vi "RT Main v0.99.vi"() -> ()   [LabVIEW 2017]
doc: "Changelog:\n\nv0.9:\n- Autocycle"
uses:
  Controls/Auto Delays.ctl
  support/Controls/All Inputs.ctl
  support/Controls/Index Details.ctl
  support/Controls/Auto Stats.ctl
  Controls/Auto Times.ctl
  Global Variables/RT GV.vi
  support/Message Queue/Enqueue Message (Single).vi
  Global Variables/FPGA GV.vi
  <vilib>/Utility/error.llb/Error Cluster From Error Code.vi
  <vilib>/rvi/errors/niLvFpgaAdjustHostInterfaceError.vi
  Global Variables/Network Globals.vi
  <vilib>/FPGAPlugInAG/Dynamic/niLvFpga_Close_Dynamic.vi
  <vilib>/rvi/interface/nirviReadWriteControl/nirviReadWriteControl.xnode
  Controls/FPGA Ref.ctl
  <vilib>/rvi/interface/nirviCloseFPGA/nirviCloseFPGA.xnode
  support/Message Queue/Message Queue.lvlib
  NiFpgaLv.dll
  <vilib>/rvi/interface/Simulation/niFpgaSimulationCallBeginRW.vi
panel:
  in  "Auto Para":T1={"Agitator Delays"=[250, 350], "TF Delays"=[700, 800, 2], "Insertion Delays"=[100, 500], "Cutting Delays"=[300, 300, 100], "PF Delays"=[250, 30000], "Measur. Delays"=[500.0, 188.9, 1.0], "Reject Delays"=[500], "BF Delays"=[1000, 1000]}
  in  "Counts in":cluster{"OutputCount":u32, "RejectCount":u32}
  in  "Stop Button 4":bool
  out "error out":errorcluster
  out "Wrong Message":string
  in  "Stop Button":bool
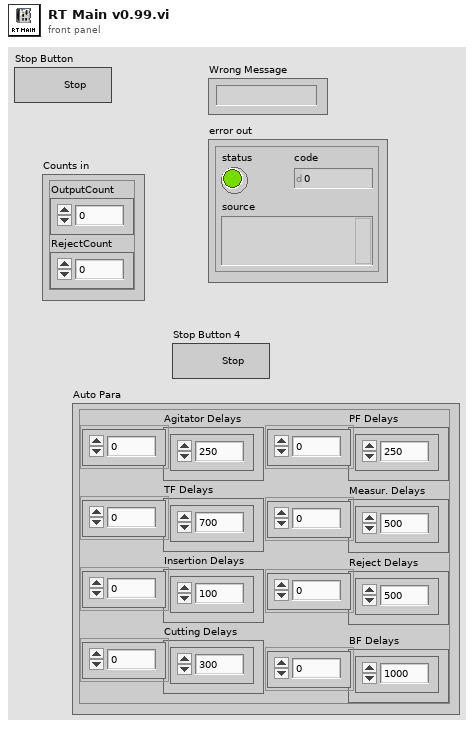
[diagram p1: front panel]
types:
  T1 = typedef "Auto Delays.ctl" = cluster{"Agitator Delays":u32[], "TF Delays":u32[], "Insertion Delays":u32[], "Cutting Delays":u32[], "PF Delays":u32[], "Measur. Delays":dbl[], "Reject Delays":u32[], "BF Delays":u32[]}
  T2 = typedef "FPGA Ref.ctl" = refnum<k20>
  T3 = cluster{"TL_Red":bool, "TL_Orange":bool, "TL_Green":bool, "TL_Buzzer":bool, "SOL_Index_Rotary_CW":bool, "SOL_Index_CNVR_Rotary_CCW":bool, "SOL_Index_CNVR_Stopper_Rear":bool, "SOL_Index_CNVR_Output _Separator _Rear":bool, "Bowl  Feeder_ ON":bool, "Pump_CNVR_Motor _ON":bool, "SOL_Gating_CYL_Rear":bool, "SOL_Tube_Feed_Agitatator":bool, "SOL_Tube_Feed_Gating_CYL":bool, "SOL_Insertion _CYL":bool, "SOL_Insertion_Clamp_CYL":bool, "SOL_Cutting_CYL":bool, "SOL_Cutting_Clamp_CYL":bool, "SOL_Insertion_Air_Nozzle":bool, "SOL_Measurement_CYL":bool, "SOL_Measure_Clamp_CYL":bool, "SOL_Rejection CYL_1":bool, "SOL_Rejection CYL_2":bool, "SOL_Rejection CYL_3":bool, "SOL_Rejection CYL_4":bool, "DO1.24":bool, "DO1.25":bool, "DO1.26":bool, "DO1.27":bool, "DO1.28":bool, "DO1.29":bool, "DO1.30":bool, "DO1.31":bool}
  T4 = typedef "All Inputs.ctl" = cluster{"DI 1":cluster{"Machine_ON":bool, "E_stop ":bool, "SW_Pressure":bool, "SW_Start ":bool, "SW_Reset":bool, "SW_Stop":bool, "SW_Door":bool, "RS_Index_Rotary_CW":bool, "RS_Index_Rotary_CCW":bool, "RS_Index_Stopper _Rear":bool, "RS_Index_Output_Separator_Rear":bool, "PES_Index_Pallet_Sensor":bool, "PES_Index_Output_Part Sensor":bool, "ICS_BF_Low_Level_1":bool, "ICS_BF_Low_Level_2":bool, "ICS_BF_Pump_CNVR_Full_1":bool, "ICS_BF_Pump_CNVR_Full_2":bool, "ICS_BF_Pump_CNVR_Full_3":bool, "ICS_BF_Pump_CNVR_Full_4":bool, "PES_PC_Pump Presence_1":bool, "PES_PC_Pump Presence_2":bool, "PES_PC_Pump Presence_3":bool, "PES_PC_Pump Presence_4":bool, "RS_PC_Gating_Front":bool, "PES_Pump_Interference":bool, "PES_TF_Low_Level":bool, "PES_Tube Presence_1":bool, "PES_Tube Presence_2":bool, "PES_Tube Presence_3":bool, "PES_Tube Presence_4":bool, "DI1.30":bool, "DI1.31":bool}, "DI 2":cluster{"RS_Agitatator_1_Rear ":bool, "RS_Agitatator_2_Rear ":bool, "RS_TF_Gating CYL_Rear":bool, "RS_Insertion_1_Rear":bool, "RS_Insertion_1_Front":bool, "RS_Insertion _2_Rear":bool, "RS_Insertion _2_Front":bool, "RS_Insertion _3_Rear":bool, "RS_Insertion _3_Front":bool, "RS_Insertion _4_Rear":bool, "RS_Insertion _4_Front":bool, "RS_Insertion_Clamp_Rear":bool, "RS_Cutting_Rear":bool, "RS_Cutting_Clamp _Rear":bool, "RS_Measurement_1_Rear":bool, "RS_Measurement_2_Rear":bool, "RS_Measurement_3_Rear":bool, "RS_Measurement_4_Rear":bool, "RS_Measure_Clamp_Rear":bool, "RS_Rejection_1_Rear":bool, "RS_Rejection_2_Rear":bool, "RS_Rejection_3_Rear":bool, "RS_Rejection_4_Rear":bool, "DI2.23":bool, "DI2.24":bool, "DI2.25":bool, "DI2.26":bool, "DI2.27":bool, "DI2.28":bool, "DI2.29":bool, "DI2.30":bool, "DI2.31":bool}, "IAS 1":dbl, "IAS 2":dbl, "IAS 3":dbl, "IAS 4":dbl, "DO 1":cluster{"TL_Red":bool, "TL_Orange":bool, "TL_Green":bool, "TL_Buzzer":bool, "SOL_Index_Rotary_CW":bool, "SOL_Index_CNVR_Rotary_CCW":bool, "SOL_Index_CNVR_Stopper_Rear":bool, "SOL_Index_CNVR_Output _Separator _Rear":bool, "Bowl  Feeder_ ON 1":bool, "Pump_CNVR_Motor _ON":bool, "SOL_PC_Gating_CYL_Rear":bool, "SOL_Tube_Feed_Agitatator":bool, "SOL_Tube_Feed_Gating_CYL":bool, "SOL_Insertion _CYL":bool, "SOL_Insertion_Clamp_CYL":bool, "SOL_Cutting_CYL":bool, "SOL_Cutting_Clamp_CYL":bool, "SOL_Insertion_Air_Nozzle":bool, "SOL_Measurement_CYL":bool, "DO1.19":bool, "SOL_Rejection CYL_1":bool, "SOL_Rejection CYL_2":bool, "SOL_Rejection CYL_3":bool, "SOL_Rejection CYL_4":bool, "Bowl  Feeder_ ON 2":bool, "SOL_BF_BlowerON":bool, "SOL_BF1_Track1":bool, "SOL_BF1_Track2":bool, "SOL_BF2_Track1":bool, "SOL_BF2_Track2":bool, "DO1.30":bool, "DO1.31":bool}}
  T5 = typedef "Index Details.ctl" = cluster{"Time (ms)":u32, "Waveform Graph":i16[]}
  T6 = cluster{T1, "Reject Pallets":cluster{"Reject 1":bool, "Reject 2":bool, "Reject 3":bool, "Reject 4":bool}}
  T7 = typedef "Auto Stats.ctl" = cluster{"Time":timestamp, "OEE":cluster{"AVL":dbl, "PRF":dbl, "QUA":dbl, "OEE":dbl}, "Auto Times":T8, "Counts out":cluster{"OutputCount":u32, "RejectCount":u32}, "Measurements":cluster{"1":dbl, "2":dbl, "3":dbl, "4":dbl}, "Outputs":cluster{"OutputCount":u32, "Numeric Control":u32}}
  T8 = typedef "Auto Times.ctl" = cluster{"Index Time":u32, "TF Time":u32, "Insertion Time":u32, "Cutting Time":u32, "PF Time":u32, "Meas. Time":u32, "Reject Time":u32}
  T9 = cluster{string, dbl, "Counts in":cluster{"OutputCount":u32, "RejectCount":u32}, "Auto Para":T1}
  T10 = cluster{"TL_Red":bool, "TL_Orange":bool, "TL_Green":bool, "TL_Buzzer":bool, "SOL_Index_Rotary_CW":bool, "SOL_Index_CNVR_Rotary_CCW":bool, "SOL_Index_CNVR_Stopper_Rear":bool, "SOL_Index_CNVR_Output _Separator _Rear":bool, "Bowl Feeder_ ON1":bool, "Pump_CNVR_Motor _ON":bool, "SOL_PC_Gating_CYL_Rear":bool, "SOL_Tube_Feed_Agitatator":bool, "SOL_Tube_Feed_Gating_CYL":bool, "SOL_Insertion _CYL":bool, "SOL_Insertion_Clamp_CYL":bool, "SOL_Cutting_CYL":bool, "SOL_Cutting_Clamp_CYL":bool, "SOL_Insertion_Air_Nozzle":bool, "SOL_Measurement_CYL":bool, "DO1.19":bool, "SOL_Rejection CYL_1":bool, "SOL_Rejection CYL_2":bool, "SOL_Rejection CYL_3":bool, "SOL_Rejection CYL_4":bool, "Bowl Feeder_ON2":bool, "SOL_BF_BlowerON":bool, "SOL_BF1_Track1":bool, "SOL_BF1_Track2":bool, "SOL_BF2_Track1":bool, "SOL_BF2_Track2":bool, "DO1.30":bool, "DO1.31":bool}
  T11 = cluster{"Machine_ON":bool, "E_stop ":bool, "SW_Pressure":bool, "SW_Start ":bool, "SW_Reset":bool, "SW_Stop":bool, "SW_Door":bool, "RS_Index_Rotary_CW":bool, "RS_Index_Rotary_CCW":bool, "RS_Index_Stopper _Rear":bool, "RS_Index_Output_Separator_Rear":bool, "PES_Index_Pallet_Sensor":bool, "PES_Index_Output_Part Sensor":bool, "ICS_BF_Low_Level_1":bool, "ICS_BF_Low_Level_2":bool, "ICS_BF_Pump_CNVR_Full_1":bool, "ICS_BF_Pump_CNVR_Full_2":bool, "ICS_BF_Pump_CNVR_Full_3":bool, "ICS_BF_Pump_CNVR_Full_4":bool, "PES_PC_Pump Presence_1":bool, "PES_PC_Pump Presence_2":bool, "PES_PC_Pump Presence_3":bool, "PES_PC_Pump Presence_4":bool, "RS_PC_Gating_Front":bool, "PES_Pump_Interference":bool, "PES_TF_Low_Level":bool, "PES_Tube Presence_1":bool, "PES_Tube Presence_2":bool, "PES_Tube Presence_3":bool, "PES_Tube Presence_4":bool, "DI1.30":bool, "DI1.31":bool}
  T12 = cluster{"RS_Agitatator_1_Rear ":bool, "RS_Agitatator_2_Rear ":bool, "RS_TF_Gating CYL_Rear":bool, "RS_Insertion_1_Rear":bool, "RS_Insertion_1_Front":bool, "RS_Insertion _2_Rear":bool, "RS_Insertion _2_Front":bool, "RS_Insertion _3_Rear":bool, "RS_Insertion _3_Front":bool, "RS_Insertion _4_Rear":bool, "RS_Insertion _4_Front":bool, "RS_Insertion_Clamp_Rear":bool, "RS_Cutting_Rear":bool, "RS_Cutting_Clamp _Rear":bool, "RS_Measurement_1_Rear":bool, "RS_Measurement_2_Rear":bool, "RS_Measurement_3_Rear":bool, "RS_Measurement_4_Rear":bool, "DI2.18":bool, "RS_Rejection_1_Rear":bool, "RS_Rejection_2_Rear":bool, "RS_Rejection_3_Rear":bool, "RS_Rejection_4_Rear":bool, "DI2.23":bool, "DI2.24":bool, "DI2.25":bool, "DI2.26":bool, "DI2.27":bool, "DI2.28":bool, "DI2.29":bool, "DI2.30":bool, "DI2.31":bool}
  T13 = cluster{"Array":string[][], "Machine Status":string}
  T14 = cluster{"Measurements":cluster{"1":dbl, "2":dbl, "3":dbl, "4":dbl}, "Reject Pallets":cluster{"Reject 1":bool, "Reject 2":bool, "Reject 3":bool, "Reject 4":bool}}
  T15 = cluster{"Auto Times":T8, "Results":cluster{"Measurements":cluster{"1":dbl, "2":dbl, "3":dbl, "4":dbl}, "Reject Pallets":cluster{"Reject 1":bool, "Reject 2":bool, "Reject 3":bool, "Reject 4":bool}}, "OutputCount":u32, "error out":errorcluster}
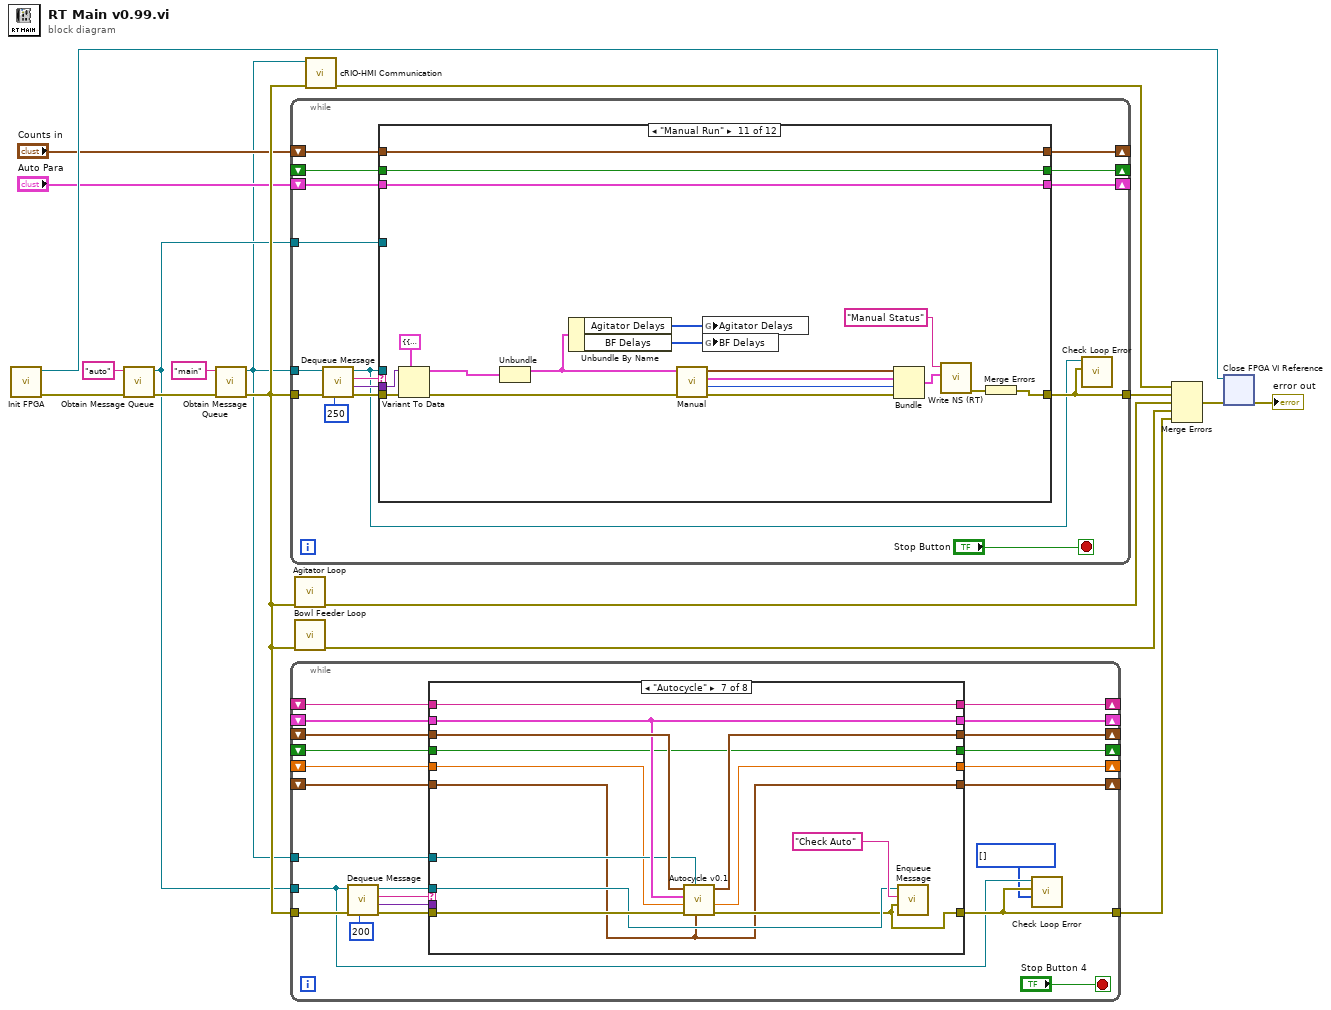
[diagram p0: block diagram]
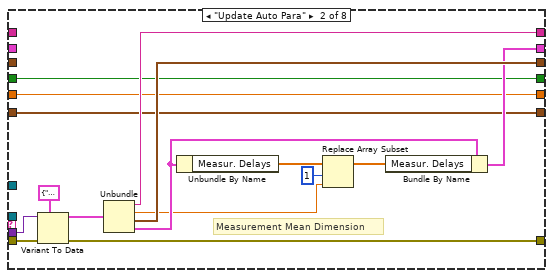
[diagram p3: hidden frame]
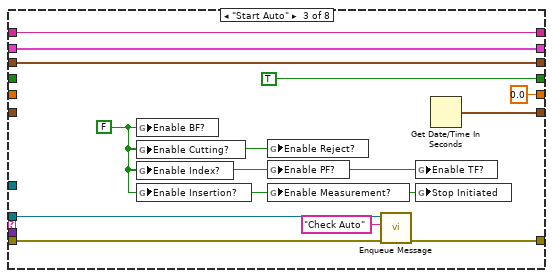
[diagram p4: hidden frame]
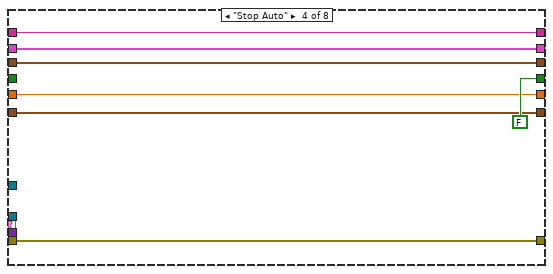
[diagram p5: hidden frame]
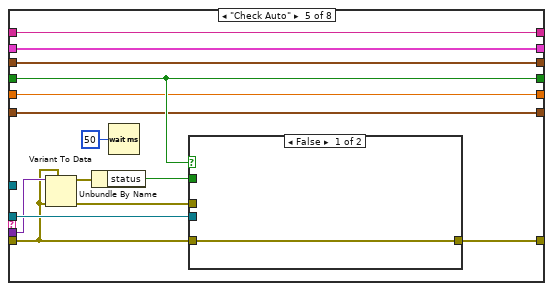
[diagram p6: hidden frame]
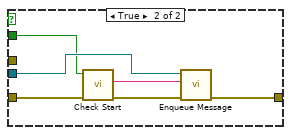
[diagram p7: hidden frame]
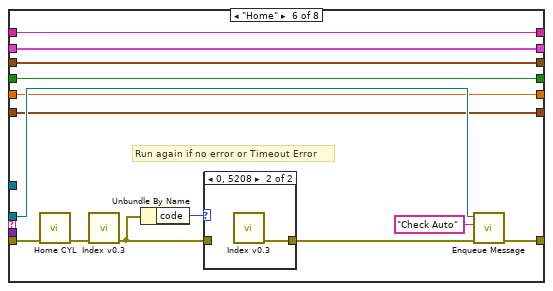
[diagram p8: hidden frame]
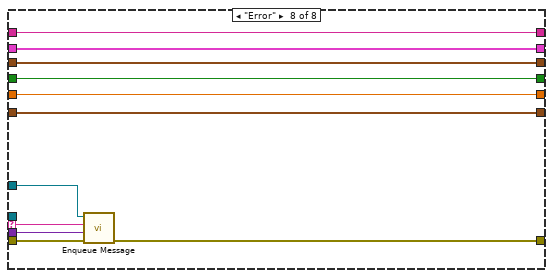
[diagram p10: hidden frame]
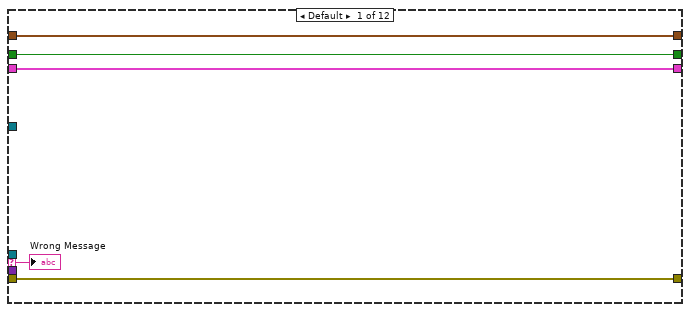
[diagram p11: hidden frame]
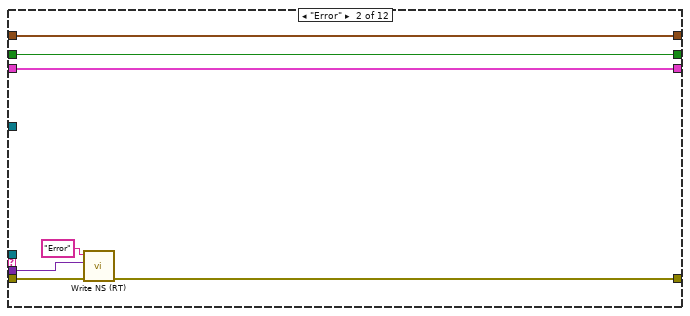
[diagram p12: hidden frame]
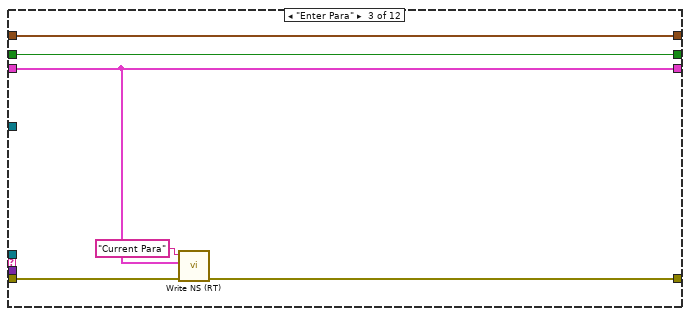
[diagram p13: hidden frame]
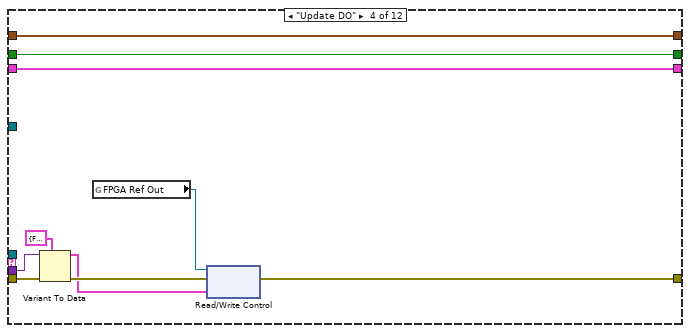
[diagram p14: hidden frame]
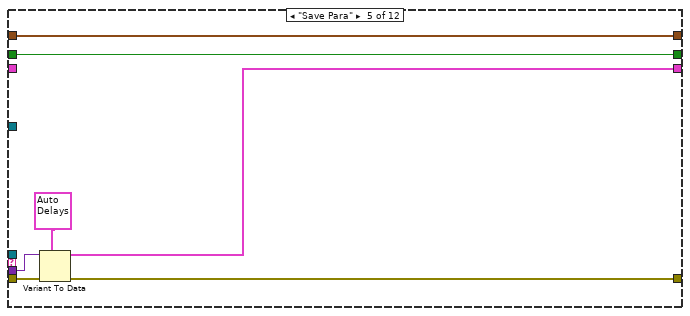
[diagram p15: hidden frame]
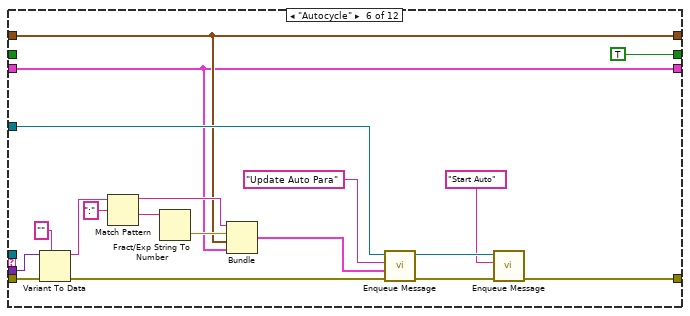
[diagram p16: hidden frame]
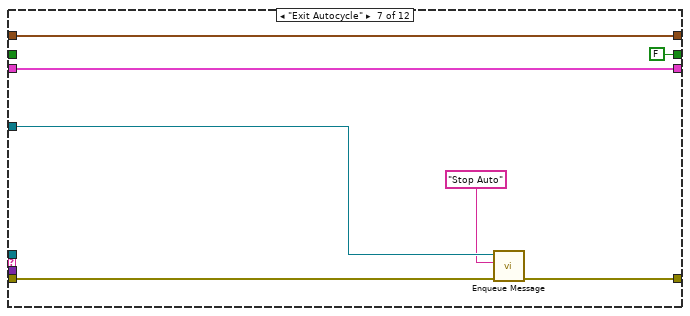
[diagram p17: hidden frame]
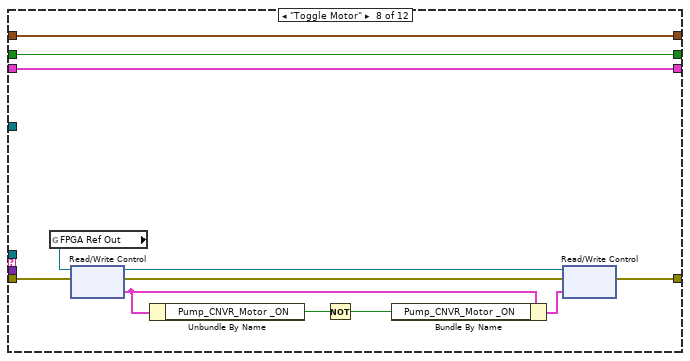
[diagram p18: hidden frame]
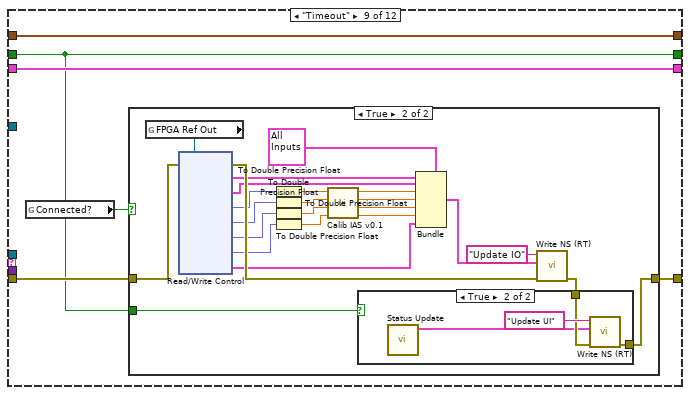
[diagram p19: hidden frame]
diagram:
  n1 = call "Init FPGA.vi"() -> ("error out"=w6:errorcluster, "FPGA Ref Out"=w11:T2)  [unwired: 10 in]
  n2 = call "Obtain Message Queue.vi"("error in (no error)"=w6, "name"="auto") -> ("error out"=w5:errorcluster, "Message Queue"=w2:refnum<queue>)  [unwired: 8 in]
  n3 = call "Obtain Message Queue.vi"("error in (no error)"=w5, "name"="main") -> ("error out"=w10:errorcluster, "Message Queue"=w1:refnum<queue>)  [unwired: 8 in]
  n4 = while {
    tunnel: w10 -> [w32]
    tunnel: w1 -> [w31]
    tunnel: [w27] -> w17
    tunnel: w2 -> [w24]
    shift-right: [w21] -> _
    shift-left: "Auto Para" -> [w22]
    shift-right: [w20] -> _
    shift-left: "Counts in" -> [w23]
    shift-right: [w18] -> _
    shift-left: _ -> [w19]
    stop <- "Stop Button" stop-if-true
    n5 = call "Dequeue Message.vi"("timeout"=250, "error in (no error)"=w32, "Message Queue"=w31) -> ("error out"=w30:errorcluster, "Message Data"=w28:variant, "Message"=w29:string, "dup Message Queue"=w26:refnum<queue>)  [unwired: 5 in]
    n6 = case shown="\"Manual Run\"" w29 {
      selector: w29 -> [w38 _ _ _ _ _ _ _ _ _ _ _]
      tunnel: w30 -> [w37 w43 w51 w61 w68 w87 w94 w105 w111 w155 w183 w194]
      tunnel: w26 -> [_ _ _ _ _ _ _ _ _ w147 _ _]
      tunnel: w28 -> [_ w41 _ w60 w67 w86 _ _ _ _ w182 w193]
      tunnel: [w37 w42 w50 w56 w66 w72 w90 w103 w112 w148 w178 w190] -> w27
      tunnel: w24 -> [_ _ _ _ _ w79 w93 _ _ _ _ _]
      tunnel: w23 -> [w36 w45 w48 w54 w65 w76 w92 w97 w109 w144 w169 w189]
      tunnel: w22 -> [w35 w44 w47 w53 _ w75 w91 w96 w108 w145 w168 w188]
      tunnel: [w35 w44 w47 w53 w64 w75 w91 w96 w108 w145 w168 w188] -> w21
      tunnel: [w36 w45 w48 w54 w65 w76 w92 w97 w109 w144 w169 w189] -> w20
      tunnel: w19 -> [w34 w39 w46 w52 w62 _ _ w95 w107 w143 w165 w184]
      tunnel: [w34 w39 w46 w52 w62 TRUE FALSE w95 w107 w143 w165 w184] -> w18
      frame Default {
        "Wrong Message" <- w38
      }
      frame "Error" {
        n7 = call "Write NS (RT).vi"("error in (no error)"=w43, "Message Data"=w41, "Message"="Error") -> ("error out"=w42:errorcluster)  [unwired: 8 in]
      }
      frame "Enter Para" {
        n8 = call "Write NS (RT).vi"("error in (no error)"=w51, "Message Data"=w47, "Message"="Current Para") -> ("error out"=w50:errorcluster)  [unwired: 8 in]
      }
      frame "Update DO" {
        n9 = Variant To Data(error in=w61, type=T3 {"TL_Red"=FALSE, "TL_Orange"=FALSE, "TL_Green"=FALSE, "TL_Buzzer"=FALSE, "SOL_Index_Rotary_CW"=FALSE, "SOL_Index_CNVR_Rotary_CCW"=FALSE, "SOL_Index_CNVR_Stopper_Rear"=FALSE, "SOL_Index_CNVR_Output _Separator _Rear"=FALSE, "Bowl  Feeder_ ON"=FALSE, "Pump_CNVR_Motor _ON"=FALSE, "SOL_Gating_CYL_Rear"=FALSE, "SOL_Tube_Feed_Agitatator"=FALSE, "SOL_Tube_Feed_Gating_CYL"=FALSE, "SOL_Insertion _CYL"=FALSE, "SOL_Insertion_Clamp_CYL"=FALSE, "SOL_Cutting_CYL"=FALSE, "SOL_Cutting_Clamp_CYL"=FALSE, "SOL_Insertion_Air_Nozzle"=FALSE, "SOL_Measurement_CYL"=FALSE, "SOL_Measure_Clamp_CYL"=FALSE, "SOL_Rejection CYL_1"=FALSE, "SOL_Rejection CYL_2"=FALSE, "SOL_Rejection CYL_3"=FALSE, "SOL_Rejection CYL_4"=FALSE, "DO1.24"=FALSE, "DO1.25"=FALSE, "DO1.26"=FALSE, "DO1.27"=FALSE, "DO1.28"=FALSE, "DO1.29"=FALSE, "DO1.30"=FALSE, "DO1.31"=FALSE} ("DO 1"), Variant=w60) -> (data=w55:T3, error out=w57:errorcluster)
        n10 = global read "FPGA GV.vi" "FPGA Ref Out"() -> (w58:T2)
        n11 = xnode "Read/Write Control"("FPGA VI Reference In"=w58, "error in"=w57, "DO 1"=w55) -> ("error out"=w56:errorcluster)  [unwired: 1 out]
      }
      frame "Save Para" {
        n12 = Variant To Data(error in=w68, type=T1 {"Agitator Delays"=[700, 250], "TF Delays"=[700, 800, 2], "Insertion Delays"=[100, 500], "Cutting Delays"=[300, 300, 100], "PF Delays"=[250, 30000], "Measur. Delays"=[500.0, 188.9, 1.0], "Reject Delays"=[500], "BF Delays"=[1000, 1000]} ("Auto Para"), Variant=w67) -> (data=w64:T1, error out=w66:errorcluster)
      }
      frame "Autocycle" {
        n13 = Variant To Data(error in=w87, type="", Variant=w86) -> (data=w82:string, error out=w80:errorcluster)
        n14 = Match Pattern(string=w82, regular expression=":") -> (before substring=w78:string, after substring=w83:string)  [unwired: 1 in, 2 out]
        n15 = Fract/Exp String To Number(string=w83) -> (number=w77:dbl)  [unwired: 3 in, 1 out]
        n16 = Bundle(w78, w77, "Counts in"=w76, "Auto Para"=w75) -> (w74:T9)  [unwired: 1 in]
        n17 = call-poly "Enqueue Message.vi"("error in (no error)"=w80, "Message Data"=w74, "Message"="Update Auto Para", "Message Queue"=w79) -> ("error out"=w73:errorcluster, "dup Message Queue"=w71:refnum<queue>)  [unwired: 6 in]
        n18 = call-poly "Enqueue Message.vi"("error in (no error)"=w73, "Message"="Start Auto", "Message Queue"=w71) -> ("error out"=w72:errorcluster)  [unwired: 7 in, 1 out]
      }
      frame "Exit Autocycle" {
        n19 = call-poly "Enqueue Message.vi"("error in (no error)"=w94, "Message"="Stop Auto", "Message Queue"=w93) -> ("error out"=w90:errorcluster)  [unwired: 7 in, 1 out]
      }
      frame "Toggle Motor" {
        n20 = global read "FPGA GV.vi" "FPGA Ref Out"() -> (w106:T2)
        n21 = xnode "Read/Write Control"("FPGA VI Reference In"=w106, "error in"=w105) -> ("FPGA VI Reference Out"=w102:T2, "error out"=w104:errorcluster, "DO 1"=w100:T10)
        n22 = Unbundle By Name(w100) -> ("Pump_CNVR_Motor _ON"=w101:bool)
        n23 = Not(x=w101) -> (.not. x?=w98:bool)
        n24 = Bundle By Name(cluster=w100, "Pump_CNVR_Motor _ON"=w98) -> (w99:T10)
        n25 = xnode "Read/Write Control"("FPGA VI Reference In"=w102, "error in"=w104, "DO 1"=w99) -> ("error out"=w103:errorcluster)  [unwired: 1 out]
      }
      frame "Timeout" {
        n26 = global read "Network Globals.vi" "Connected?"() -> (w110:bool)
        n27 = case shown="True" w110 {
          tunnel: [w113 w116] -> w112
          tunnel: w111 -> [w113 w136]
          tunnel: w107 -> [_ w114]
          frame False {
          }
          frame True {
            n28 = global read "FPGA GV.vi" "FPGA Ref Out"() -> (w115:T2)
            n29 = xnode "Read/Write Control"("FPGA VI Reference In"=w115, "error in"=w136) -> ("error out"=w135:errorcluster, "DI 1"=w134:T11, "DI 2"=w133:T12, "AI0"=w132:fxp<+/-,27,6>, "AI1"=w131:fxp<+/-,27,6>, "AI2"=w130:fxp<+/-,27,6>, "AI3"=w129:fxp<+/-,27,6>, "DO 1"=w126:T10)  [unwired: 1 out]
            n30 = To Double Precision Float(number=w132) -> (double precision float=w119:dbl)
            n31 = To Double Precision Float(number=w131) -> (double precision float=w121:dbl)
            n32 = To Double Precision Float(number=w130) -> (double precision float=w123:dbl)
            n33 = To Double Precision Float(number=w129) -> (double precision float=w125:dbl)
            n34 = call "Calib IAS v0.1.vi"("x 4"=w125, "x 3"=w123, "x 2"=w121, "x"=w119) -> ("y 4"=w124:dbl, "y 3"=w122:dbl, "y 2"=w120:dbl, "y 1"=w118:dbl)  [unwired: 2 in, 2 out]
            n35 = Bundle(cluster=T4 {"DI 1"={"Machine_ON"=FALSE, "E_stop "=FALSE, "SW_Pressure"=FALSE, "SW_Start "=FALSE, "SW_Reset"=FALSE, "SW_Stop"=FALSE, "SW_Door"=FALSE, "RS_Index_Rotary_CW"=FALSE, "RS_Index_Rotary_CCW"=FALSE, "RS_Index_Stopper _Rear"=FALSE, "RS_Index_Output_Separator_Rear"=FALSE, "PES_Index_Pallet_Sensor"=FALSE, "PES_Index_Output_Part Sensor"=FALSE, "ICS_BF_Low_Level_1"=FALSE, "ICS_BF_Low_Level_2"=FALSE, "ICS_BF_Pump_CNVR_Full_1"=FALSE, "ICS_BF_Pump_CNVR_Full_2"=FALSE, "ICS_BF_Pump_CNVR_Full_3"=FALSE, "ICS_BF_Pump_CNVR_Full_4"=FALSE, "PES_PC_Pump Presence_1"=FALSE, "PES_PC_Pump Presence_2"=FALSE, "PES_PC_Pump Presence_3"=FALSE, "PES_PC_Pump Presence_4"=FALSE, "RS_PC_Gating_Front"=FALSE, "PES_Pump_Interference"=FALSE, "PES_TF_Low_Level"=FALSE, "PES_Tube Presence_1"=FALSE, "PES_Tube Presence_2"=FALSE, "PES_Tube Presence_3"=FALSE, "PES_Tube Presence_4"=FALSE, "DI1.30"=FALSE, "DI1.31"=FALSE}, "DI 2"={"RS_Agitatator_1_Rear "=FALSE, "RS_Agitatator_2_Rear "=FALSE, "RS_TF_Gating CYL_Rear"=FALSE, "RS_Insertion_1_Rear"=FALSE, "RS_Insertion_1_Front"=FALSE, "RS_Insertion _2_Rear"=FALSE, "RS_Insertion _2_Front"=FALSE, "RS_Insertion _3_Rear"=FALSE, "RS_Insertion _3_Front"=FALSE, "RS_Insertion _4_Rear"=FALSE, "RS_Insertion _4_Front"=FALSE, "RS_Insertion_Clamp_Rear"=FALSE, "RS_Cutting_Rear"=FALSE, "RS_Cutting_Clamp _Rear"=FALSE, "RS_Measurement_1_Rear"=FALSE, "RS_Measurement_2_Rear"=FALSE, "RS_Measurement_3_Rear"=FALSE, "RS_Measurement_4_Rear"=FALSE, "RS_Measure_Clamp_Rear"=FALSE, "RS_Rejection_1_Rear"=FALSE, "RS_Rejection_2_Rear"=FALSE, "RS_Rejection_3_Rear"=FALSE, "RS_Rejection_4_Rear"=FALSE, "DI2.23"=FALSE, "DI2.24"=FALSE, "DI2.25"=FALSE, "DI2.26"=FALSE, "DI2.27"=FALSE, "DI2.28"=FALSE, "DI2.29"=FALSE, "DI2.30"=FALSE, "DI2.31"=FALSE}, "IAS 1"=0.0, "IAS 2"=0.0, "IAS 3"=0.0, "IAS 4"=0.0, "DO 1"={"TL_Red"=FALSE, "TL_Orange"=FALSE, "TL_Green"=FALSE, "TL_Buzzer"=FALSE, "SOL_Index_Rotary_CW"=FALSE, "SOL_Index_CNVR_Rotary_CCW"=FALSE, "SOL_Index_CNVR_Stopper_Rear"=FALSE, "SOL_Index_CNVR_Output _Separator _Rear"=FALSE, "Bowl  Feeder_ ON 1"=FALSE, "Pump_CNVR_Motor _ON"=FALSE, "SOL_PC_Gating_CYL_Rear"=FALSE, "SOL_Tube_Feed_Agitatator"=FALSE, "SOL_Tube_Feed_Gating_CYL"=FALSE, "SOL_Insertion _CYL"=FALSE, "SOL_Insertion_Clamp_CYL"=FALSE, "SOL_Cutting_CYL"=FALSE, "SOL_Cutting_Clamp_CYL"=FALSE, "SOL_Insertion_Air_Nozzle"=FALSE, "SOL_Measurement_CYL"=FALSE, "DO1.19"=FALSE, "SOL_Rejection CYL_1"=FALSE, "SOL_Rejection CYL_2"=FALSE, "SOL_Rejection CYL_3"=FALSE, "SOL_Rejection CYL_4"=FALSE, "Bowl  Feeder_ ON 2"=FALSE, "SOL_BF_BlowerON"=FALSE, "SOL_BF1_Track1"=FALSE, "SOL_BF1_Track2"=FALSE, "SOL_BF2_Track1"=FALSE, "SOL_BF2_Track2"=FALSE, "DO1.30"=FALSE, "DO1.31"=FALSE}}, "DI 1"=w134, "DI 2"=w133, "IAS 1"=w118, "IAS 2"=w120, "IAS 3"=w122, "IAS 4"=w124, "DO 1"=w126) -> (w128:T4)
            n36 = call "Write NS (RT).vi"("error in (no error)"=w135, "Message Data"=w128, "Message"="Update IO") -> ("error out"=w117:errorcluster)  [unwired: 8 in]
            n37 = case shown="True" w114 {
              tunnel: w117 -> [w138 w141]
              tunnel: [w138 w140] -> w116
              frame False {
              }
              frame True {
                n38 = call "Status Update.vi"() -> ("Status Cluster"=w139:T13)  [unwired: 11 in]
                n39 = call "Write NS (RT).vi"("error in (no error)"=w141, "Message Data"=w139, "Message"="Update UI") -> ("error out"=w140:errorcluster)  [unwired: 8 in]
              }
            }
          }
        }
      }
      frame "Manual Index" {
        n40 = call "Index v0.3.vi"("error in (no error)"=w155) -> ("error out"=w153:errorcluster, "Waveform Graph"=w151:i16[], "Index Time"=w152:u32)  [unwired: 7 in, 1 out]
        n41 = Bundle(cluster=T5 {"Time (ms)"=0, "Waveform Graph"=[]}, "Time (ms)"=w152, "Waveform Graph"=w151) -> (w150:T5)
        n42 = call "Write NS (RT).vi"("error in (no error)"=w153, "Message Data"=w150, "Message"="Update Index") -> ("error out"=w149:errorcluster)  [unwired: 8 in]
        n43 = flat-sequence {
          tunnel: w149 -> [w159]
          tunnel: [w158] -> w148
          tunnel: w147 -> [w156]
          frame #0 {
            n44 = global read "RT GV.vi" "Continuous Index?"() -> (w157:bool)
            n45 = case shown="True" w157 {
              tunnel: w159 -> [w160 w164]
              tunnel: [w160 w163] -> w158
              tunnel: w156 -> [_ w161]
              frame False {
              }
              frame True {
                n46 = call-poly "Enqueue Message.vi"("error in (no error)"=w164, "Message"="Manual Index", "Message Queue"=w161) -> ("error out"=w163:errorcluster)  [unwired: 7 in, 1 out]
              }
            }
          }
        }
      }
      frame "Manual Run" {
        n47 = Variant To Data(error in=w183, type=T6 {{"Agitator Delays"=[1000], "TF Delays"=[1000], "Insertion Delays"=[1000], "Cutting Delays"=[1000], "PF Delays"=[1000], "Measur. Delays"=[1000.0], "Reject Delays"=[1000], "BF Delays"=[1000]}, "Reject Pallets"={"Reject 1"=FALSE, "Reject 2"=FALSE, "Reject 3"=FALSE, "Reject 4"=FALSE}}, Variant=w182) -> (data=w174:T6, error out=w181:errorcluster)
        n48 = Unbundle(w174) -> (w171:T1)  [unwired: 1 out]
        n49 = Unbundle By Name(w171) -> ("Agitator Delays"=w167:u32[], "BF Delays"=w166:u32[])
        n50 = call "Manual.vi"("error in"=w181, "Auto Delays"=w171) -> ("error out"=w173:errorcluster, "OutputCount"=w172:u32, "Results"=w170:T14, "Auto Times"=w177:T8)  [unwired: 6 in]
        n51 = global write "RT GV.vi" "Agitator Delays"(w167) -> ()
        n52 = global write "RT GV.vi" "BF Delays"(w166) -> ()
        n53 = Bundle("Auto Times"=w177, "Results"=w170, "OutputCount"=w172, "error out"=w173) -> (w176:T15)  [unwired: 1 in]
        n54 = call "Write NS (RT).vi"("Message Data"=w176, "Message"="Manual Status") -> ("error out"=w179:errorcluster)  [unwired: 9 in]
        n55 = Merge Errors(w179) -> (w178:errorcluster)
      }
      frame "Log Cycle" {
        n56 = Variant To Data(error in=w194, type=T7 {"Time"=timestamp(0 s since 1904-01-01), "OEE"={"AVL"=100.0, "PRF"=100.0, "QUA"=100.0, "OEE"=0.0}, "Auto Times"={"Index Time"=0, "TF Time"=0, "Insertion Time"=0, "Cutting Time"=0, "PF Time"=0, "Meas. Time"=0, "Reject Time"=0}, "Counts out"={"OutputCount"=0, "RejectCount"=0}, "Measurements"={"1"=0.0, "2"=0.0, "3"=0.0, "4"=0.0}, "Outputs"={"OutputCount"=0, "Numeric Control"=0}} ("Auto Stats"), Variant=w193) -> (data=w185:T7, error out=w186:errorcluster)
        n57 = call "Write NS (RT).vi"("error in (no error)"=w186, "Message Data"=w185, "Message"="Autocycle Log") -> ("error out"=w191:errorcluster)  [unwired: 8 in]
        n58 = Merge Errors(w191) -> (w190:errorcluster)
      }
    }
    n59 = call "Check Loop Error.vi"("error to process"=w27, "Message Queue"=w26) -> ()  [unwired: 8 in, 2 out]
  }
  n60 = while {
    tunnel: w10 -> [w213]
    tunnel: [w211] -> w9
    shift-right: [w215] -> _
    shift-left: _ -> [w216]
    tunnel: w2 -> [w203]
    shift-right: [w207] -> _
    shift-left: _ -> [w206]
    shift-right: [w205] -> _
    shift-left: _ -> [w204]
    shift-right: [w202] -> _
    shift-left: _ -> [w201]
    tunnel: w1 -> [w200]
    shift-right: [w198] -> _
    shift-left: _ -> [w197]
    shift-right: [w196] -> _
    shift-left: _ -> [w195]
    stop <- "Stop Button 4" stop-if-true
    n61 = call "Dequeue Message.vi"("timeout"=200, "error in (no error)"=w213, "Message Queue"=w203) -> ("error out"=w212:errorcluster, "Message Data"=w208:variant, "Message"=w209:string, "dup Message Queue"=w210:refnum<queue>)  [unwired: 5 in]
    n62 = case shown="\"Autocycle\"" w209 {
      selector: w209 -> [_ _ _ _ _ _ _ w315]
      tunnel: w212 -> [w224 w240 w247 w255 w263 w289 w308 w313]
      tunnel: [w224 w239 w246 w255 w269 w284 w299 w312] -> w211
      tunnel: w216 -> [w223 _ w251 w258 w272 w293 w307 w319]
      tunnel: [w223 w234 w251 w258 w272 w293 w306 w319] -> w215
      tunnel: w210 -> [_ _ w245 _ w268 w282 w300 _]
      tunnel: w208 -> [_ w238 _ _ w265 _ _ w314]
      tunnel: [w222 w235 w250 w257 w271 w292 w305 w318] -> w207
      tunnel: w206 -> [w222 _ w250 w257 w271 w292 w305 w318]
      tunnel: [w221 w228 w249 w256 w270 w291 w304 w317] -> w205
      tunnel: w204 -> [w221 _ w249 w256 w270 w291 w304 w317]
      tunnel: [w220 w227 TRUE FALSE w267 w290 w302 w316] -> w202
      tunnel: w201 -> [w220 w227 _ _ w267 w290 w302 w316]
      tunnel: w200 -> [_ _ _ _ _ _ w303 w311]
      tunnel: [w218 w226 0.0 ("Run Time out") w252 w259 w280 w298 w309] -> w198
      tunnel: w197 -> [w218 w226 _ w252 w259 w280 w297 w309]
      tunnel: w195 -> [w219 w225 _ w253 w260 w281 w296 w310]
      tunnel: [w219 w225 w242 w253 w260 w281 w296 w310] -> w196
      frame Default {
      }
      frame "Update Auto Para" {
        # "Measurement Mean Dimension"
        n63 = Variant To Data(error in=w240, type=T9 {"", 0.0, "Counts in"={"OutputCount"=0, "RejectCount"=0}, "Auto Para"={"Agitator Delays"=[], "TF Delays"=[], "Insertion Delays"=[], "Cutting Delays"=[], "PF Delays"=[], "Measur. Delays"=[], "Reject Delays"=[], "BF Delays"=[]}} ("cluster"), Variant=w238) -> (data=w236:T9, error out=w239:errorcluster)
        n64 = Unbundle(w236) -> (w235:string, w230:dbl, "Counts in"=w234:cluster{"OutputCount":u32, "RejectCount":u32}, "Auto Para"=w233:T1)
        n65 = Unbundle By Name(w233) -> ("Measur. Delays"=w232:dbl[])
        n66 = Replace Array Subset(array=w232, new element=w230, index=1) -> (w229:dbl[])
        n67 = Bundle By Name(cluster=w233, "Measur. Delays"=w229) -> (w228:T1)
      }
      frame "Start Auto" {
        w243 = FALSE ("Enable BF?")
        n68 = global write "RT GV.vi" "Enable BF?"(w243) -> ()
        n69 = global write "RT GV.vi" "Enable Cutting?"(w243) -> ()
        n70 = global write "RT GV.vi" "Enable Index?"(w243) -> ()
        n71 = global write "RT GV.vi" "Enable Insertion?"(w243) -> ()
        n72 = global write "RT GV.vi" "Enable Reject?"(w243) -> ()
        n73 = global write "RT GV.vi" "Enable PF?"(w243) -> ()
        n74 = global write "RT GV.vi" "Enable Measurement?"(w243) -> ()
        n75 = call-poly "Enqueue Message.vi"("error in (no error)"=w247, "Message"="Check Auto", "Message Queue"=w245) -> ("error out"=w246:errorcluster)  [unwired: 7 in, 1 out]
        n76 = global write "RT GV.vi" "Enable TF?"(w243) -> ()
        n77 = global write "RT GV.vi" "Stop Initiated"(w243) -> ()
        n78 = Get Date/Time In Seconds() -> (seconds since 1Jan1904=w242:timestamp)
      }
      frame "Stop Auto" {
      }
      frame "Check Auto" {
        n79 = Variant To Data(error in=w263, type=w263, Variant=w265) -> (data=w262:errorcluster, error out=w264:errorcluster)
        n80 = Unbundle By Name(w262) -> ("status"=w261:bool)
        n81 = Wait (ms)(milliseconds to wait=u32 50) -> ()  [unwired: 1 out]
        n82 = case shown="False" w267 {
          tunnel: [w273 w279] -> w269
          tunnel: w268 -> [_ w275]
          tunnel: w263 -> [w273 w278]
          tunnel: w264 -> [_ _]
          tunnel: w261 -> [_ w274]
          frame False {
          }
          frame True {
            n83 = call "Check Start.vi"("error in"=w278, "Error Stop?"=w274) -> ("error out"=w277:errorcluster, "Message"=w276:string)  [unwired: 8 in]
            n84 = call-poly "Enqueue Message.vi"("error in (no error)"=w277, "Message"=w276, "Message Queue"=w275) -> ("error out"=w279:errorcluster)  [unwired: 7 in, 1 out]
          }
        }
      }
      frame "Home" {
        # "Run again if no error or Timeout Error"
        n85 = call "Home CYL.vi"("error in"=w289) -> ("error out"=w288:errorcluster)  [unwired: 10 in]
        n86 = call "Index v0.3.vi"("error in (no error)"=w288) -> ("error out"=w286:errorcluster)  [unwired: 7 in, 3 out]
        n87 = Unbundle By Name(w286) -> ("code"=w287:i32)
        n88 = case shown="0, 5208" w287 {
          tunnel: [w294 w295] -> w283
          tunnel: w286 -> [w294 _]
          frame Default {
          }
          frame 0, 5208 {
            n89 = call "Index v0.3.vi"() -> ("error out"=w295:errorcluster)  [unwired: 8 in, 3 out]
          }
        }
        n90 = call-poly "Enqueue Message.vi"("error in (no error)"=w283, "Message"="Check Auto", "Message Queue"=w282) -> ("error out"=w284:errorcluster)  [unwired: 7 in, 1 out]
      }
      frame "Autocycle" {
        n91 = call "Autocycle v0.1.vi"("start time"=w296, "Message Queue"=w303, "error in"=w308, "Run Time in"=w297, "Auto Para"=w304, "Counts in"=w307) -> ("error out"=w299:errorcluster, "Run Time out"=w298:dbl, "Counts out"=w306:cluster{"OutputCount":u32, "RejectCount":u32})  [unwired: 3 in]
        n92 = call-poly "Enqueue Message.vi"("Message Data"=w299, "Message"="Check Auto", "Message Queue"=w300) -> ()  [unwired: 7 in, 2 out]
      }
      frame "Error" {
        n93 = call-poly "Enqueue Message.vi"("error in (no error)"=w313, "Message Data"=w314, "Message"=w315, "Message Queue"=w311) -> ("error out"=w312:errorcluster)  [unwired: 6 in, 1 out]
      }
    }
    n94 = call "Check Loop Error.vi"("Ignore Errors"=i32[] [], "error to process"=w211, "Message Queue"=w203) -> ()  [unwired: 7 in, 2 out]
  }
  n95 = call "Agitator Loop.vi"("error in (no error)"=w10) -> ("error out"=w13:errorcluster)  [unwired: 10 in]
  n96 = call "Bowl Feeder Loop.vi"("error in (no error)"=w10) -> ("error out"=w12:errorcluster)  [unwired: 10 in]
  n97 = call "cRIO-HMI Communication.vi"("error in (no error)"=w10, "Message Queue"=w1) -> ("error out"=w16:errorcluster)  [unwired: 9 in]
  n98 = Merge Errors(w16, w17, w13, w12, w9) -> (w15:errorcluster)
  n99 = xnode ("Close FPGA VI Reference")("FPGA VI Reference In"=w11, "error in"=w15) -> ("error out"=→"error out":errorcluster)
